vi "is_inside.vi"(8 "error in (no error)":errorcluster, 10 "SpaceVector.lvclass":refnum<class "SpaceVector.lvclass">, 11 "Box in":refnum<class "Box.lvclass">) -> (0 "error out":errorcluster, 2 "is inside?":bool, 3 "Box out":refnum<class "Box.lvclass">)   [LabVIEW 2010, in "Box.lvclass"]
uses:
  Box.lvclass
  SpaceVector/SpaceVector/SpaceVector.lvclass
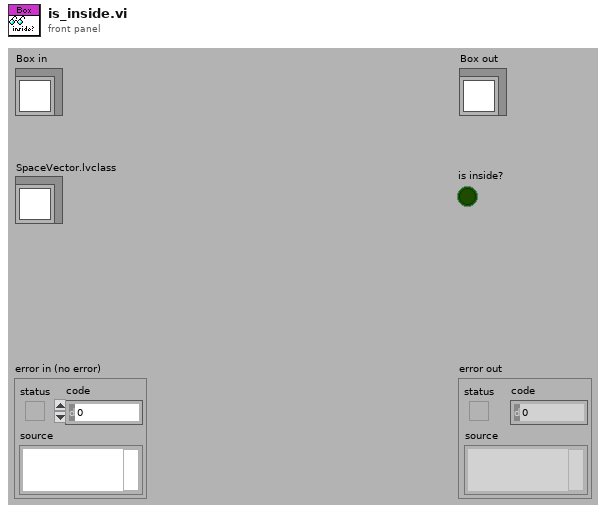
[diagram p1: front panel]
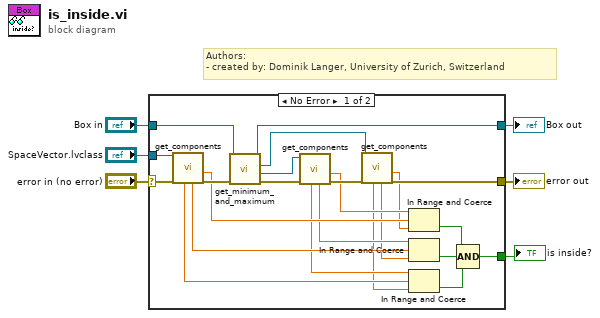
[diagram p0: block diagram]
diagram:
  # "Authors: \n- created by: Dominik Langer, University of Zurich, Switzerland"
  n1 = case shown="No Error" "error in (no error)" {
    selector: "error in (no error)" -> [w28 w31]
    tunnel: [w20 w31] -> w5
    tunnel: [w26 w30] -> w3
    tunnel: "Box in" -> [w27 w30]
    tunnel: "SpaceVector.lvclass" -> [w29 _]
    tunnel: [w7 _] -> w1
    frame No Error {
      n2 = call "get_components.vi"("error in (no error)"=w28, "SpaceVector in"=w29) -> ("error out"=w25:errorcluster, "x"=w19:dbl[unit], "z"=w15:dbl[unit], "y"=w16:dbl[unit])  [unwired: 4 in, 2 out]
      n3 = call "get_minimum_and_maximum.vi"("error in (no error)"=w25, "Box in"=w27) -> ("error out"=w22:errorcluster, "maximum"=w23:refnum<class "SpaceVector.lvclass">, "minimum"=w24:refnum<class "SpaceVector.lvclass">, "Box out"=w26:refnum<class "Box.lvclass">)  [unwired: 6 in]
      n4 = call "get_components.vi"("error in (no error)"=w22, "SpaceVector in"=w23) -> ("error out"=w21:errorcluster, "x"=w18:dbl[unit], "z"=w14:dbl[unit], "y"=w12:dbl[unit])  [unwired: 4 in, 2 out]
      n5 = call "get_components.vi"("error in (no error)"=w21, "SpaceVector in"=w24) -> ("error out"=w20:errorcluster, "x"=w17:dbl[unit], "z"=w13:dbl[unit], "y"=w11:dbl[unit])  [unwired: 4 in, 2 out]
      n6 = In Range and Coerce(upper limit=w18, x=w19, lower limit=w17) -> (In Range?=w10:bool)  [unwired: 1 out]
      n7 = In Range and Coerce(upper limit=w14, x=w15, lower limit=w13) -> (In Range?=w9:bool)  [unwired: 1 out]
      n8 = In Range and Coerce(upper limit=w12, x=w16, lower limit=w11) -> (In Range?=w8:bool)  [unwired: 1 out]
      n9 = Compound Arithmetic op=AND(w10, w9, w8) -> (w7:bool)
    }
    frame Error {
    }
  }
  "error out" <- w5
  "Box out" <- w3
  "is inside?" <- w1
